vi "Determine Warnings.vi"() -> ()   [LabVIEW 2014]
panel:
  out "Warning?":bool
  out "Warning Text":string
  in  "Min Temp":dbl
  in  "Max Temp":dbl
  in  "Current Temp":dbl
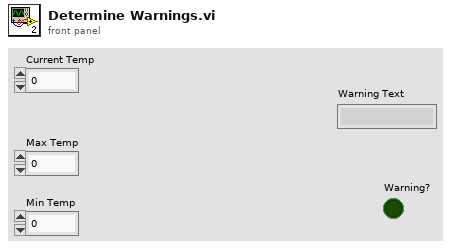
[diagram p1: front panel]
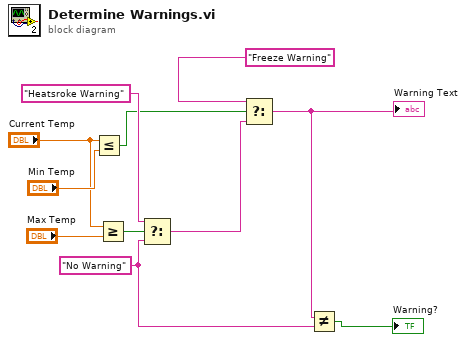
[diagram p0: block diagram]
diagram:
  w3 = "No Warning"
  n1 = Less Or Equal?(x="Current Temp", y="Min Temp") -> (x <= y?=w6:bool)
  n2 = Greater Or Equal?(x="Current Temp", y="Max Temp") -> (x >= y?=w8:bool)
  n3 = Select(t="Heatsroke Warning", s=w8, f=w3) -> (s? t:f=w4:string)
  n4 = Select(t="Freeze Warning", s=w6, f=w4) -> (s? t:f=w1:string)
  "Warning Text" <- w1
  n5 = Not Equal?(x=w1, y=w3) -> (x != y?=→"Warning?":bool)
